vi "Midi_convert.vi"(11 "read":string) -> (3 "current value":dbl, 5 "ble?":bool)   [LabVIEW 2022 SP3]
panel:
  out "array":dbl[](array[numeric])
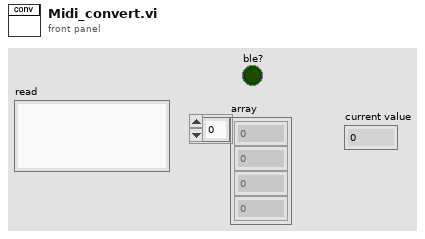
[diagram p1: front panel]
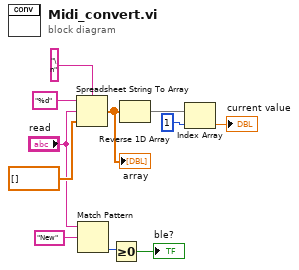
[diagram p0: block diagram]
diagram:
  n1 = Spreadsheet String To Array(delimiter (Tab)="\n", format string="%d", spreadsheet string="read", array type (2D Dbl)=dbl[] []) -> (array=w6:dbl[])
  "array" <- w6
  n2 = Match Pattern(string="read", regular expression="New") -> (offset past match=w2:i32)  [unwired: 1 in, 3 out]
  n3 = Greater Or Equal To 0?(x=w2) -> (x >= 0?=→"ble?":bool)
  n4 = Reverse 1D Array(array=w6) -> (reversed array=w5:dbl[])
  n5 = Index Array(array=w5, index=1) -> (element=→"current value":dbl)
